vi "Filter Error Codes (Scalar)__ogtk.vi"(4 "Upstream Error (optional)":errorcluster, 8 "Error In":errorcluster, 10 "Error Code to Filter":i32) -> (0 "Error Out":errorcluster, 1 "Error Filtered?":bool, 2 "Filtered Error Details":T1)   [LabVIEW 2012]
doc: "Filters <b>Error In</b> if matches <b>Error Code to Filter</b>. An <b>Upstream Error</b> can be optionally merged with the resulting filtered error."
uses:
  <userlib>/_OpenG.lib/error/error.llb/Filtered Error Details - Cluster__ogtk.ctl
panel:
  # "Please visit http://www.OpenG.org to learn about the\nOpen Source LabVIEW software movement.\n\nNOTICE -- YOU MUST LEAVE THIS NOTICE IN PLACE.  PER THE TERMS OF THE LICENSE BELOW, YOU MAY SUBLICENSE THIS SOFTWARE \nIN ANY WAY THAT DOES NOT CONFLICT WITH THIS LICENSE.\n\n### BSD License (http://www.opensource.org/licenses/bsd-license.php) Begin ###\n \nCopyright (c) 2011, JKI <info@jki.net>\nCopyright (c) 2011, Jonathon Green <jg@jgcode.net>\n\nAll rights reserved.\n\nRedistribution and use in source and binary forms, with or without modification, are permitted provided that the following conditions are met:\n\n    * Redistributions of source code must retain the above copyright notice, this list of conditions and the following disclaimer.\n    * Redistributions in binary form must reproduce the above copyright notice, this list of conditions and the following disclaimer in the \n       documentation and/or other materials provided with the distribution.\n    * Neither the name of SciWare, James Kring, Inc., nor the names of its contributors may be used to endorse or promote products derived \n       from this software without specific prior written permission.\n\nTHIS SOFTWARE IS PROVIDED BY THE COPYRIGHT HOLDERS AND CONTRIBUTORS \"AS IS\" AND ANY EXPRESS OR IMPLIED WARRANTIES, \nINCLUDING, BUT NOT LIMITED TO, THE IMPLIED WARRANTIES OF MERCHANTABILITY AND FITNESS FOR A PARTICULAR PURPOSE ARE \nDISCLAIMED. IN NO EVENT SHALL THE COPYRIGHT OWNER OR CONTRIBUTORS BE LIABLE FOR ANY DIRECT, INDIRECT, INCIDENTAL,\n SPECIAL, EXEMPLARY, OR CONSEQUENTIAL DAMAGES (INCLUDING, BUT NOT LIMITED TO, PROCUREMENT OF SUBSTITUTE GOODS OR \nSERVICES; LOSS OF USE, DATA, OR PROFITS; OR BUSINESS INTERRUPTION) HOWEVER CAUSED AND ON ANY THEORY OF LIABILITY, \nWHETHER IN CONTRACT, STRICT LIABILITY, OR TORT (INCLUDING NEGLIGENCE OR OTHERWISE) ARISING IN ANY WAY OUT OF THE USE \nOF THIS SOFTWARE, EVEN IF ADVISED OF THE POSSIBILITY OF SUCH DAMAGE.\n\n### BSD License End ###"
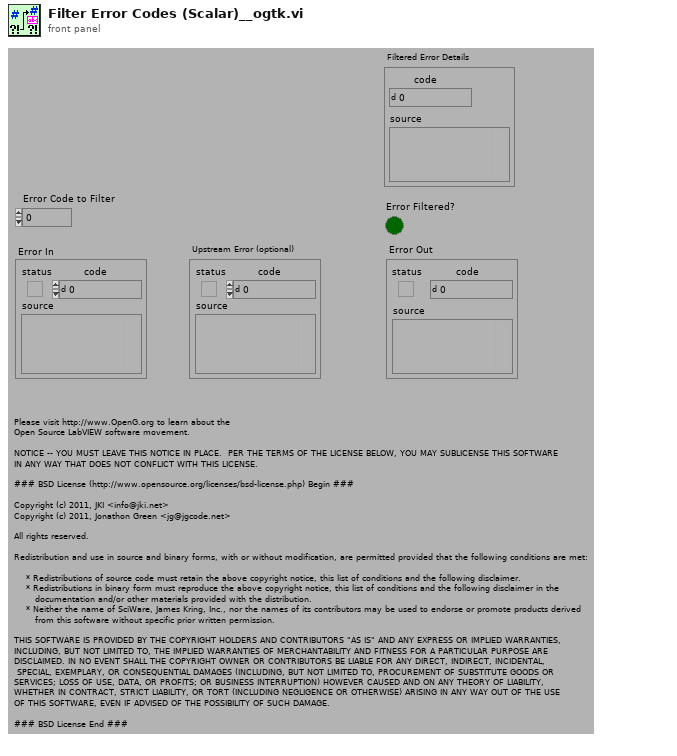
[diagram p1: front panel]
types:
  T1 = typedef "Filtered Error Details - Cluster__ogtk.ctl" = cluster{"code":i32, "source":string}
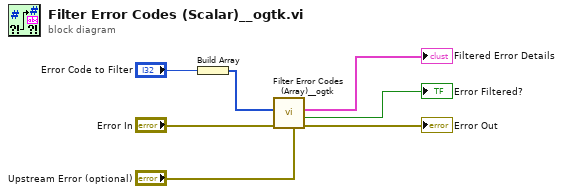
[diagram p0: block diagram]
diagram:
  n1 = Build Array("Error Code to Filter") -> (w4:i32[])
  n2 = call <userlib>:"Filter Error Codes (Array)__ogtk.vi"("Upstream Error (optional)"="Upstream Error (optional)", "Error In"="Error In", "Error Codes to Filter"=w4) -> ("Error Out"=→"Error Out":errorcluster, "Error Filtered?"=→"Error Filtered?":bool, "Filtered Error Details"=→"Filtered Error Details":T1)  [unwired: 6 in]
